vi "ChoosePass.vi"(8 "error in (no error)":errorcluster, 9 "Enum":enum16{"Striker", "2ndStriker"}(ring), 10 "Game":refnum<class "Game.lvclass">, 11 "Utilities in":refnum<class "Utilities.lvclass">) -> (0 "error out":errorcluster, 2 "Result":dbl, 3 "Utilities out":refnum<class "Utilities.lvclass">)   [LabVIEW 2018, in "Utilities.lvclass"]
uses:
  Utilities.lvclass
  Game_class/Game.lvclass
  Robot_class/roles.ctl
  Game_class/Game.lvclass/Game.ctl
  Team_class/Team.lvclass/Team.ctl
  Object_class/Object.lvclass/Object.ctl
  Robot_class/Robot.lvclass/Robot.ctl
  Referee_class/Referee.lvclass/Referee.ctl
  Object_class/Read x.vi
  Object_class/Read y.vi
  Robot_class/Read role.vi
  Robot_class/Read id.vi
  ef69b4df-9ac6-409c-8cda-008bb4cff728.vi
  Referee_class/Read enemy_goalie_id.vi
  Team_class/Read RobotRef.vi
  Game_class/Read OffensiveTeam.vi
  Game_class/Read BallRef.vi
  Game_class/Read FieldRef.vi
  Game_class/Read EnemyRef.vi
  Game_class/Read Referee.vi
  <vilib>/Array/Sort 2D Array - Pop Stack.vi
  <vilib>/Array/Sort 2D Array - Push Stack.vi
  Ally_class/Ally.lvclass
  C:/Users/Felipe/Desktop/Nova pasta/SSL_AI/Team_class/Team.lvclass
  Robot_class/Robot.lvclass
  C:/Users/Felipe/Desktop/Nova pasta/SSL_AI/Object_class/Object.lvclass
  Enemy_class/Enemy.lvclass
  Ball_class/Ball.lvclass
  Field_class/Field.lvclass
  Referee_class/Referee.lvclass
panel:
  in  "y5":dbl=0.07
  in  "y4":dbl=0.16
  in  "y3":dbl=0.4
  in  "y2":dbl=0.17
  in  "y":dbl=0.2
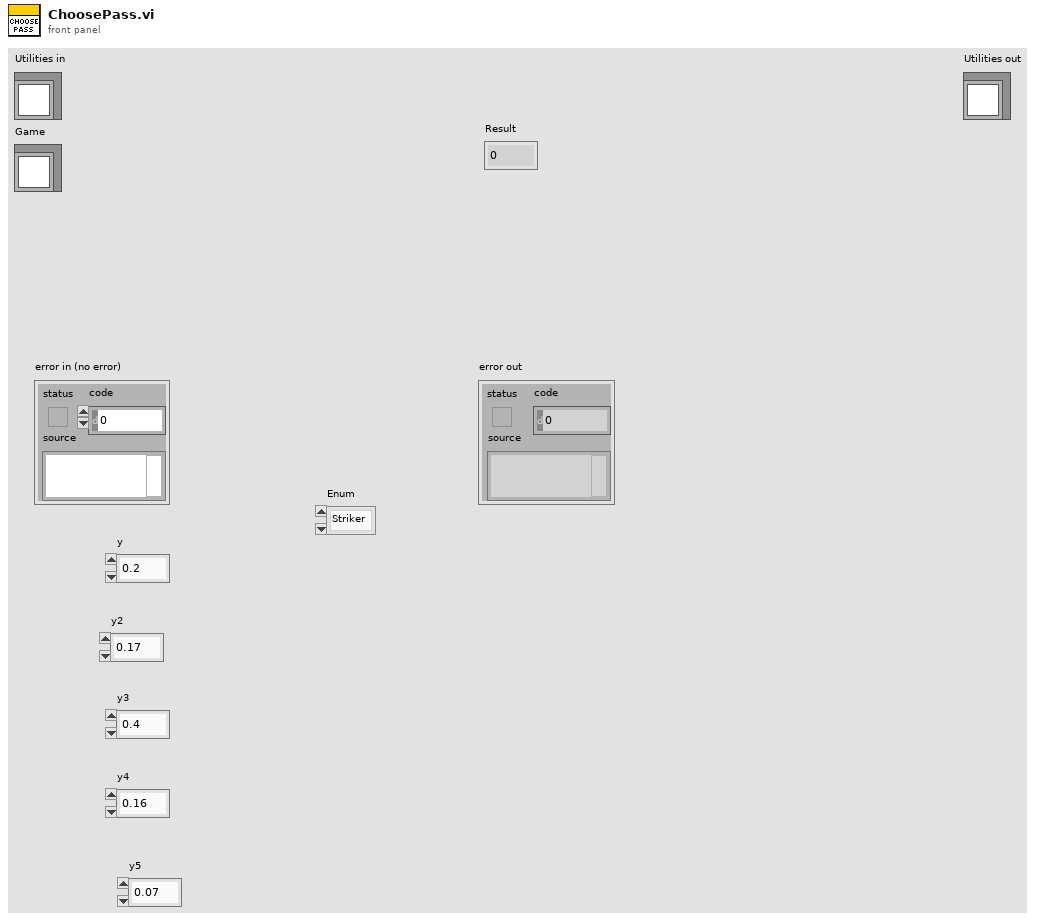
[diagram p1: front panel]
types:
  T1 = typedef "roles.ctl" = enum16{"PenaltyDefense", "PreparePassReceiver", "PassObserver", "Timeout", "Goto", "ZigZag", "None", "BallOutOfField", "DefenderArea", "Duelist", "AttackerStop", "FollowAttacker", "KeeperRole", "KickPenalty", "AttackerAimGoal", "AttackerBlock", "Marker", "Halt", "Shoot", "PassKicker", "PassReceiver", "TestRole", "PenaltyAttacker"}
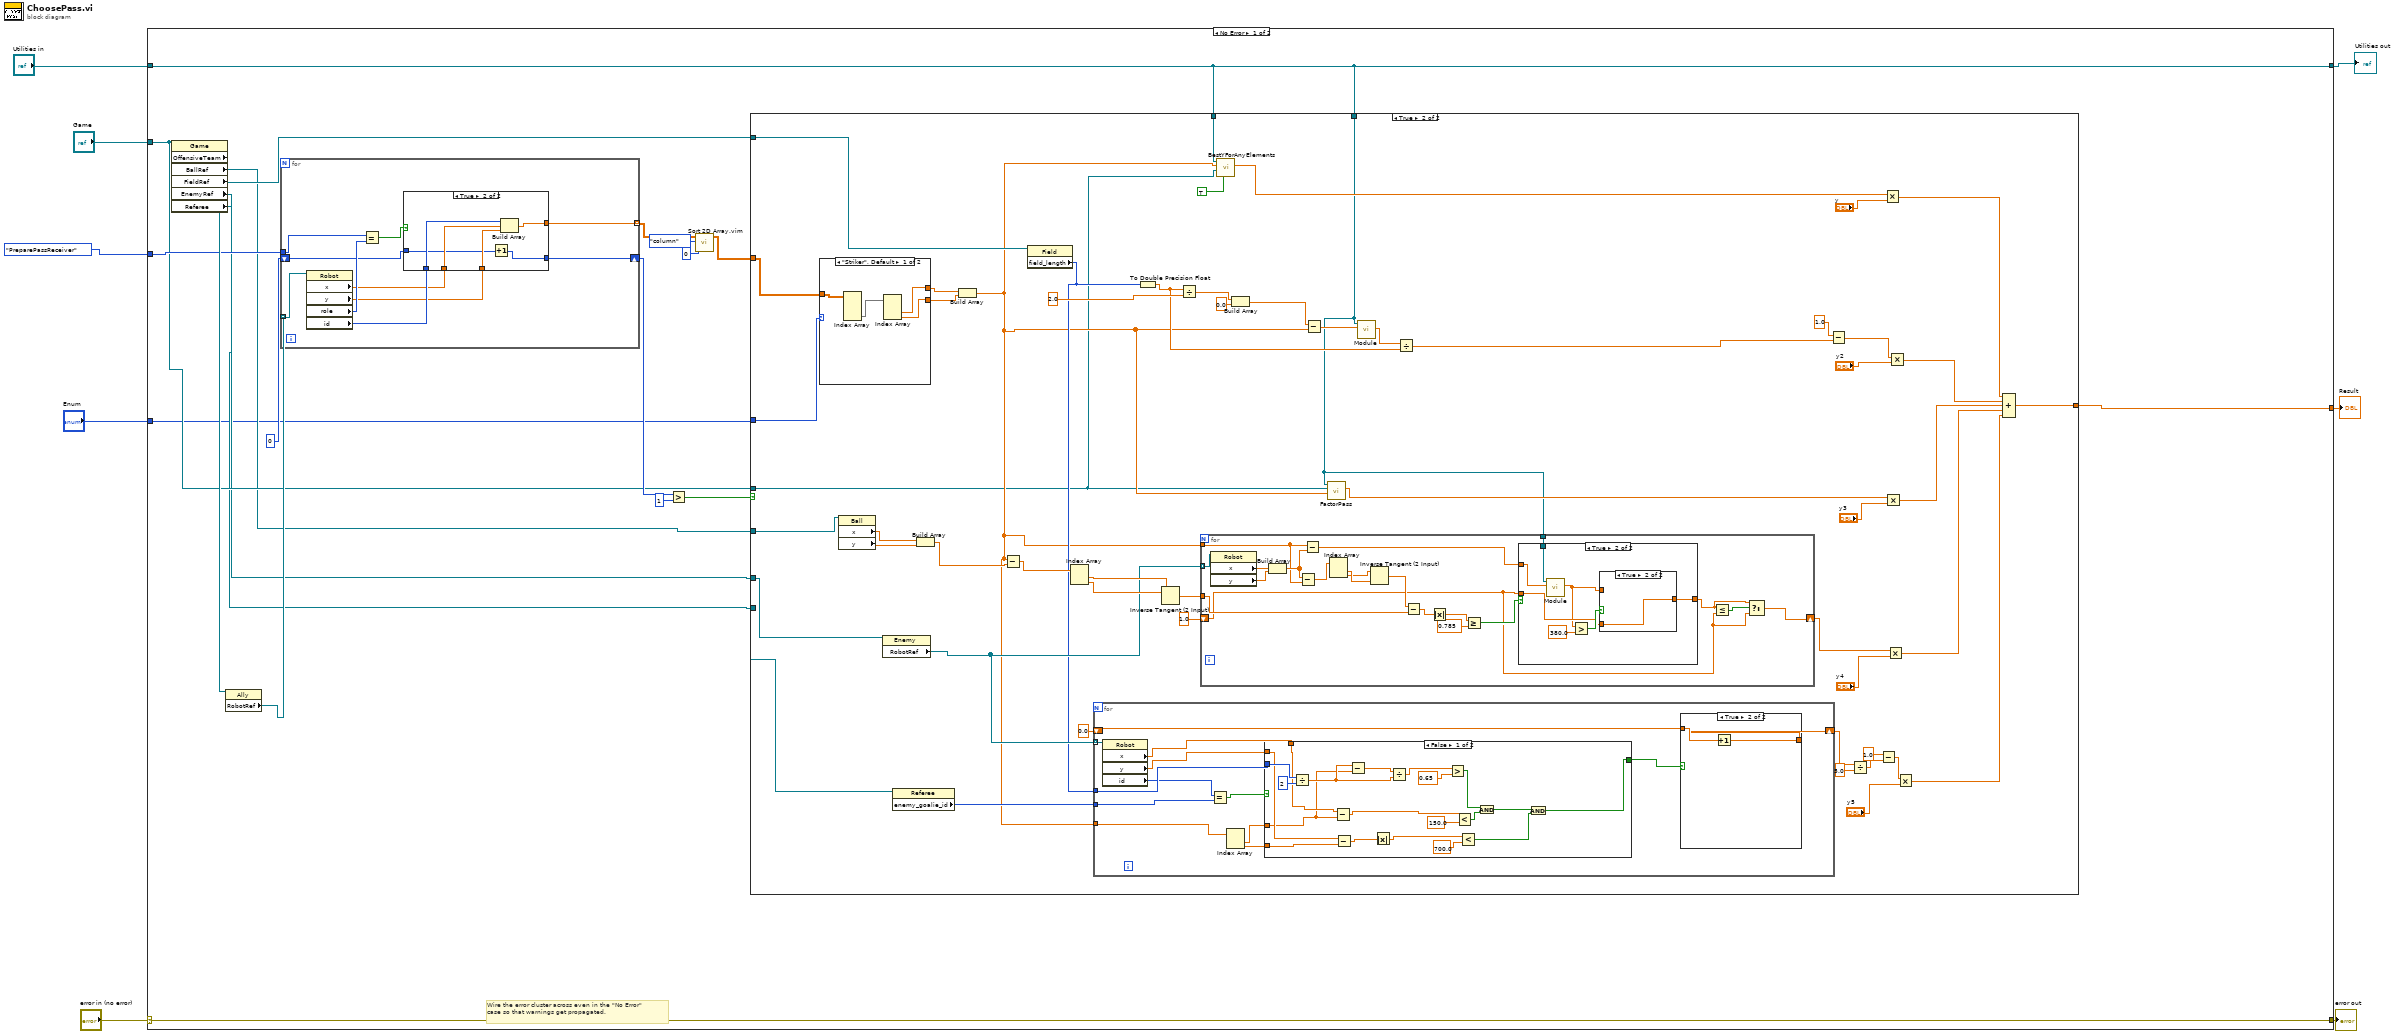
[diagram p0: block diagram]
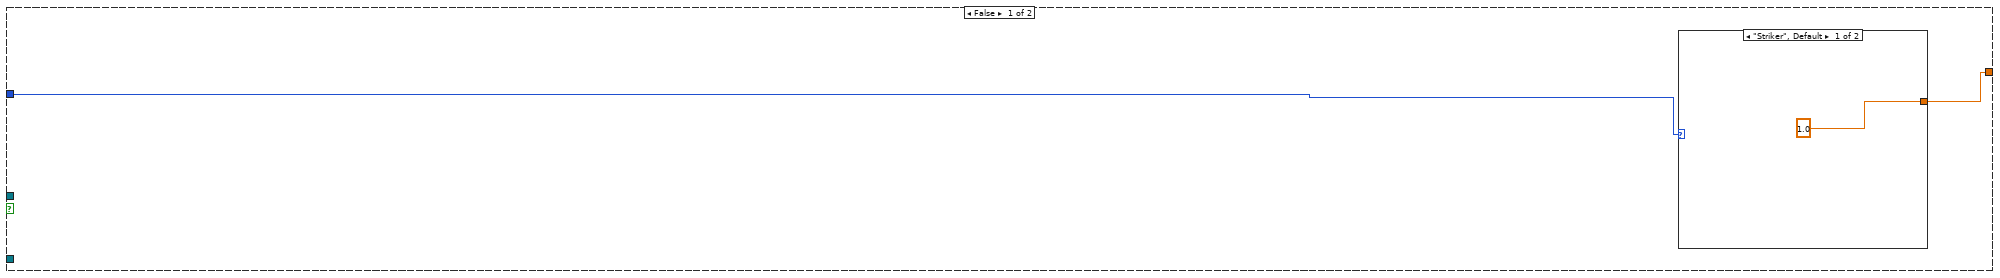
[diagram p2: hidden frame]
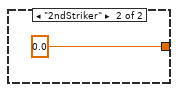
[diagram p3: hidden frame]
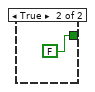
[diagram p4: hidden frame]
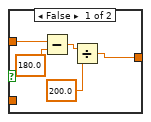
[diagram p7: hidden frame]
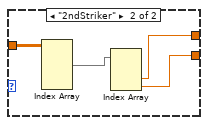
[diagram p8: hidden frame]
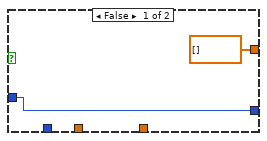
[diagram p9: hidden frame]
diagram:
  n1 = case shown="No Error" "error in (no error)" {
    selector: "error in (no error)" -> [w28 w185]
    tunnel: [w28 w185] -> w7
    tunnel: "Game" -> [w15 _]
    tunnel: roles."PreparePassReceiver" ("x") -> [w16 _]
    tunnel: [w11 _] -> w4
    tunnel: "Utilities in" -> [w10 w184]
    tunnel: [w10 w184] -> w2
    tunnel: "Enum" -> [w9 _]
    frame No Error {
      # "Wire the error cluster across even in the \"No Error\"\ncase so that warnings get propagated."
      n2 = property class="Game"(reference=w15) -> ("OffensiveTeam"=w27:refnum<class "Ally.lvclass">, "BallRef"=w14:refnum<class "Ball.lvclass">, "FieldRef"=w17:refnum<class "Field.lvclass">, "EnemyRef"=w13:refnum<class "Enemy.lvclass">, "Referee"=w12:refnum<class "Referee.lvclass">)  [unwired: 1 in, 2 out]
      n3 = property class="Ally"(reference=w27) -> ("RobotRef"=w26:refnum<class "Robot.lvclass">[])  [unwired: 1 in, 2 out]
      n4 = for {
        tunnel: w26 -> [w175] mode=indexing
        shift-right: [w168] -> w21
        shift-left: 0 -> [w169]
        tunnel: [w167] -> w24 mode=indexing
        tunnel: w16 -> [w166]
        n5 = property class="Robot"(reference=w175) -> ("x"=w171:dbl, "y"=w170:dbl, "role"=w174:T1, "id"=w173:i32)  [unwired: 1 in, 2 out]
        n6 = Equal?(x=w166, y=w174) -> (x = y?=w172:bool)
        n7 = case shown="True" w172 {
          tunnel: w173 -> [_ w181]
          tunnel: w171 -> [_ w183]
          tunnel: w170 -> [_ w182]
          tunnel: w169 -> [w176 w180]
          tunnel: [w176 w179] -> w168
          tunnel: [dbl[] [] w178] -> w167
          frame False {
          }
          frame True {
            n8 = Increment(x=w180) -> (x+1=w179:i32)
            n9 = Build Array(w181, w183, w182) -> (w178:dbl[])
          }
        }
      }
      n10 = Greater?(x=w21, y=1) -> (0:w19:bool)
      n11 = call "Sort 2D Array.vim"("index"=0, "dimension to index (column)"=enum16{"column", "row"}."column", "2D array"=w24) -> ("sorted 2D array"=w18:dbl[][])  [unwired: 7 in, 1 out]
      n12 = case shown="True" w19 {
        tunnel: w18 -> [_ w86]
        tunnel: w9 -> [w30 w85]
        tunnel: w17 -> [_ w82]
        tunnel: w15 -> [_ w37]
        tunnel: w14 -> [_ w62]
        tunnel: w13 -> [_ w54]
        tunnel: w12 -> [_ w53]
        tunnel: [w29 w39] -> w11
        tunnel: w10 -> [_ w34]
        tunnel: w10 -> [_ w33]
        frame False {
          n13 = case shown="\"Striker\", Default" w30 {
            tunnel: [1.0 0.0] -> w29
            frame "Striker", Default {
            }
            frame "2ndStriker" {
            }
          }
        }
        frame True {
          n14 = case shown="\"Striker\", Default" w85 {
            tunnel: w86 -> [w161 w165]
            tunnel: [w159 w163] -> w84
            tunnel: [w158 w162] -> w83
            frame "Striker", Default {
              n15 = Index Array(array=w161) -> (element #2=w160:dbl[])  [unwired: 4 in, 1 out]
              n16 = Index Array(array=w160) -> (element #2=w159:dbl, element #3=w158:dbl)  [unwired: 3 in, 1 out]
            }
            frame "2ndStriker" {
              n17 = Index Array(array=w165) -> (element #1=w164:dbl[])  [unwired: 4 in, 1 out]
              n18 = Index Array(array=w164) -> (element #2=w163:dbl, element #3=w162:dbl)  [unwired: 3 in, 1 out]
            }
          }
          n19 = property class="Ball"(reference=w62) -> ("x"=w61:dbl, "y"=w60:dbl)  [unwired: 1 in, 2 out]
          n20 = property class="Enemy"(reference=w54) -> ("RobotRef"=w42:refnum<class "Robot.lvclass">[])  [unwired: 1 in, 2 out]
          n21 = property class="Referee"(reference=w53) -> ("enemy_goalie_id"=w41:i32)  [unwired: 1 in, 2 out]
          n22 = Build Array(w61, w60) -> (w59:dbl[])
          n23 = Build Array(w84, w83) -> (w38:dbl[])
          n24 = Subtract(x=w38, y=w59) -> (x-y=w58:dbl[])
          n25 = property class="Field"(reference=w82) -> ("field_length"=w40:i32)  [unwired: 1 in, 2 out]
          n26 = Index Array(array=w58) -> (element #1=w56:dbl, element #2=w57:dbl)  [unwired: 2 in]
          n27 = for {
            tunnel: w38 -> [w93]
            shift-right: [w98] -> w48
            shift-left: 0.0 -> [w99]
            tunnel: w41 -> [w97]
            tunnel: w40 -> [w94]
            tunnel: w42 -> [w90] mode=indexing
            n28 = property class="Robot"(reference=w90) -> ("x"=w88:dbl, "y"=w87:dbl, "id"=w89:i32)  [unwired: 1 in, 2 out]
            n29 = Equal?(x=w89, y=w97) -> (x = y?=w96:bool)
            n30 = Index Array(array=w93) -> (element #1=w92:dbl, element #2=w91:dbl)  [unwired: 2 in]
            n31 = case shown="False" w96 {
              tunnel: [w101 FALSE] -> w95
              tunnel: w94 -> [w119 _]
              tunnel: w88 -> [w112 _]
              tunnel: w92 -> [w100 _]
              tunnel: w87 -> [w110 _]
              tunnel: w91 -> [w109 _]
              frame False {
                n32 = Divide(x=w119, y=u32 2) -> (x/y=w116:dbl)
                n33 = Subtract(x=w112, y=w100) -> (x-y=w111:dbl)
                n34 = Subtract(x=w110, y=w109) -> (x-y=w108:dbl)
                n35 = Subtract(x=w116, y=w100) -> (x-y=w117:dbl)
                n36 = Absolute Value(x=w108) -> (abs(x)=w107:dbl)
                n37 = Divide(x=w117, y=w116) -> (x/y=w115:dbl)
                n38 = Greater?(x=w115, y=0.65) -> (0:w105:bool)
                n39 = Less?(x=w111, y=150.0) -> (x < y?=w104:bool)
                n40 = Less?(x=w107, y=700.0) -> (x < y?=w102:bool)
                n41 = And(x=w105, y=w104) -> (x .and. y?=w103:bool)
                n42 = And(x=w103, y=w102) -> (x .and. y?=w101:bool)
              }
              frame True {
              }
            }
            n43 = case shown="True" w95 {
              tunnel: w99 -> [w121 w123]
              tunnel: [w121 w122] -> w98
              frame False {
              }
              frame True {
                n44 = Increment(x=w123) -> (x+1=w122:dbl)
              }
            }
          }
          n45 = To Double Precision Float(number=w40) -> (double precision float=w73:dbl)
          n46 = Inverse Tangent (2 Input)(1:w56, 2:w57) -> (0:w55:dbl)
          n47 = Divide(x=w73, y=2.0) -> (x/y=w80:dbl)
          n48 = for {
            tunnel: w55 -> [w138]
            tunnel: w38 -> [w125]
            tunnel: w42 -> [w134] mode=indexing
            shift-right: [w127] -> w52
            shift-left: 1.0 ("element") -> [w126]
            tunnel: w34 -> [w124]
            n49 = property class="Robot"(reference=w134) -> ("x"=w133:dbl, "y"=w132:dbl)  [unwired: 1 in, 2 out]
            n50 = Build Array(w133, w132) -> (w131:dbl[])
            n51 = Subtract(x=w131, y=w125) -> (x-y=w143:dbl[])
            n52 = Subtract(x=w125, y=w131) -> (x-y=w130:dbl[])
            n53 = Index Array(array=w143) -> (element #1=w140:dbl, element #2=w139:dbl)  [unwired: 2 in]
            n54 = Inverse Tangent (2 Input)(1:w140, 2:w139) -> (0:w142:dbl)
            n55 = Subtract(x=w142, y=w138) -> (x-y=w141:dbl)
            n56 = Absolute Value(x=w141) -> (abs(x)=w136:dbl)
            n57 = Greater Or Equal?(x=w136, y=0.785) -> (x >= y?=w135:bool)
            n58 = case shown="True" w135 {
              tunnel: w126 -> [w144 w147]
              tunnel: w130 -> [_ w151]
              tunnel: [w144 w149] -> w128
              tunnel: w124 -> [_ w145]
              frame False {
              }
              frame True {
                n59 = call-dynamic "Module.vi"("2D vector"=w151, "Utilities in"=w145) -> ("Modulo"=w146:dbl)  [unwired: 7 in, 2 out]
                n60 = Greater?(x=w146, y=380.0) -> (0:w148:bool)
                n61 = case shown="True" w148 {
                  tunnel: w147 -> [_ w157]
                  tunnel: [w156 w157] -> w149
                  tunnel: w146 -> [w155 _]
                  frame False {
                    n62 = Subtract(x=w155, y=180.0) -> (x-y=w153:dbl)
                    n63 = Divide(x=w153, y=200.0) -> (x/y=w156:dbl)
                  }
                  frame True {
                  }
                }
              }
            }
            n64 = Less Or Equal?(x=w128, y=w126) -> (x <= y?=w129:bool)
            n65 = Select(t=w128, s=w129, f=w126) -> (s? t:f=w127:dbl)
          }
          n66 = call "BestYForAnyElements.vi"("Boolean"=TRUE, "Game"=w37, "Array"=w38, "Utilities in"=w33) -> ("Goal gap"=w35:dbl)  [unwired: 5 in, 2 out]
          n67 = Build Array(w80, 0.0 ("element")) -> (w78:dbl[])
          n68 = Subtract(x=w78, y=w38) -> (x-y=w77:dbl[])
          n69 = call-dynamic "FactorPass.vi"("Coordenada robo"=w38, "Game"=w37, "Utilities in"=w34) -> ("Critério de marcação Normalizado"=w63:dbl)  [unwired: 6 in, 2 out]
          n70 = call-dynamic "Module.vi"("2D vector"=w77, "Utilities in"=w34) -> ("Modulo"=w76:dbl)  [unwired: 7 in, 2 out]
          n71 = Divide(x=w76, y=w73) -> (x/y=w75:dbl)
          n72 = Subtract(x=1.0, y=w75) -> (x-y=w72:dbl)
          n73 = Divide(x=w48, y=5.0) -> (x/y=w46:dbl)
          n74 = Subtract(x=1.0, y=w46) -> (x-y=w44:dbl)
          n75 = Multiply(x=w35, y="y") -> (x*y=w70:dbl)
          n76 = Multiply(x=w63, y="y3") -> (x*y=w67:dbl)
          n77 = Multiply(x=w52, y="y4") -> (x*y=w66:dbl)
          n78 = Multiply(x=w72, y="y2") -> (x*y=w71:dbl)
          n79 = Multiply(x=w44, y="y5") -> (x*y=w49:dbl)
          n80 = Compound Arithmetic op=ADD(w70, w71, w67, w66, w49) -> (w39:dbl)
        }
      }
    }
    frame Error {
    }
  }
  "error out" <- w7
  "Result" <- w4
  "Utilities out" <- w2
